vi "MoveToAbsolutePosition.vi"(0 "axis in":cluster{"keyHandle":u32, "nodeId":u16}={"keyHandle"=0, "nodeId"=1}, 5 "position profile":T1, 7 "absolute position":i32, 9 "timeout":u32, 11 "error in (no error)":errorcluster) -> (4 "axis out":cluster{"keyHandle":u32, "nodeId":u16}={"keyHandle"=0, "nodeId"=1}, 15 "error out":errorcluster)   [LabVIEW 2018]
doc: "<B>MoveToAbsolutePosition</B> starts immediately an absolute positioning. Before the positioning starts, the position profile is written."
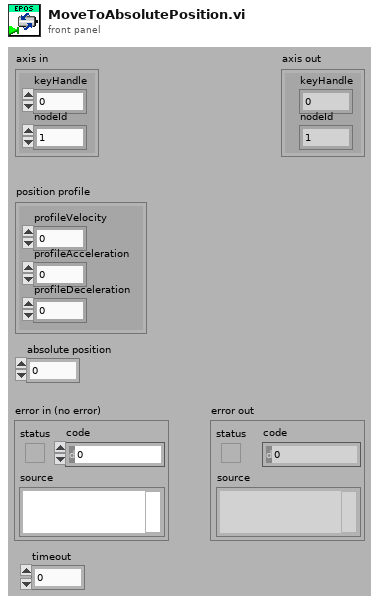
[diagram p1: front panel]
types:
  T1 = cluster{"profileVelocity":u32, "profileAcceleration":u32, "profileDeceleration":u32}
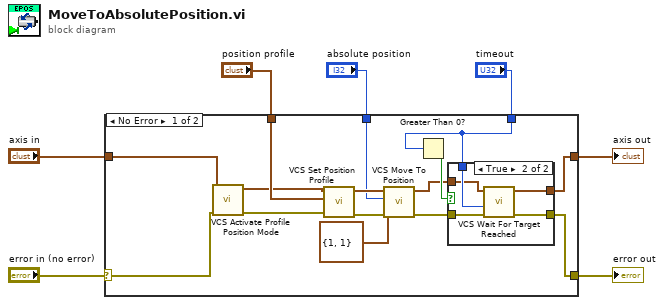
[diagram p0: block diagram]
diagram:
  n1 = case shown="No Error" "error in (no error)" {
    selector: "error in (no error)" -> [w8 w31]
    tunnel: [w13 w31] -> w6
    tunnel: [w14 w30] -> w5
    tunnel: "axis in" -> [w9 w30]
    tunnel: "position profile" -> [w20 _]
    tunnel: "absolute position" -> [w19 _]
    tunnel: "timeout" -> [w16 _]
    frame No Error {
      n2 = call "VCS Activate Profile Position Mode.vi"("error in (no error)"=w8, "axis in"=w9) -> ("error out"=w11:errorcluster, "axis out"=w10:cluster{"keyHandle":u32, "nodeId":u16})  [unwired: 8 in]
      n3 = call "VCS Set Position Profile.vi"("error in (no error)"=w11, "position profile"=w20, "axis in"=w10) -> ("error out"=w21:errorcluster, "axis out"=w22:cluster{"keyHandle":u32, "nodeId":u16})  [unwired: 7 in]
      n4 = call "VCS Move To Position.vi"("error in (no error)"=w21, "flags"=cluster{"Absolute":i32, "Immediately":i32} {"Absolute"=1, "Immediately"=1}, "targetPosition"=w19, "axis in"=w22) -> ("error out"=w12:errorcluster, "axis out"=w15:cluster{"keyHandle":u32, "nodeId":u16})  [unwired: 6 in]
      n5 = Greater Than 0?(x=w16) -> (x > 0?=w17:bool)
      n6 = case shown="True" w17 {
        tunnel: w16 -> [_ w29]
        tunnel: w15 -> [w24 w28]
        tunnel: [w24 w27] -> w14
        tunnel: [w23 w26] -> w13
        tunnel: w12 -> [w23 w25]
        frame False {
        }
        frame True {
          n7 = call "VCS Wait For Target Reached.vi"("error in (no error)"=w25, "timeout"=w29, "axis in"=w28) -> ("error out"=w26:errorcluster, "axis out"=w27:cluster{"keyHandle":u32, "nodeId":u16})  [unwired: 7 in]
        }
      }
    }
    frame Error {
    }
  }
  "error out" <- w6
  "axis out" <- w5
